vi "OFDM Symbol Type Mapper.vi"(9 "format":enum16{"NON_HT_OFDM", "VHT", "NON_HT_DUP_OFDM"}(ring), 10 "OFDM symbol index":u16) -> (2 "Cluster":T1)   [LabVIEW 2020]
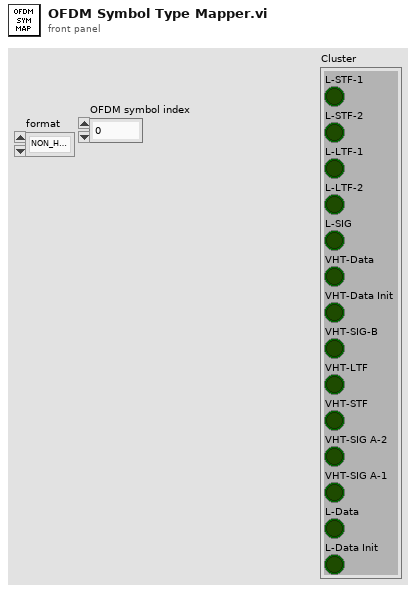
[diagram p1: front panel]
types:
  T1 = cluster{"L-STF-1":bool, "L-STF-2":bool, "L-LTF-1":bool, "L-LTF-2":bool, "L-SIG":bool, "VHT-Data":bool, "VHT-Data Init":bool, "VHT-SIG-B":bool, "VHT-LTF":bool, "VHT-STF":bool, "VHT-SIG A-2":bool, "VHT-SIG A-1":bool, "L-Data":bool, "L-Data Init":bool}
  T2 = enum16{"L-STF-1", "L-STF-2", "L-LTF-1", "L-LTF-2", "L-SIG", "L-Data-Init", "L-Data", "VHT-SIG A-1", "VHT-SIG A-2", "VHT-STF", "VHT-LTF", "VHT-SIG-B", "VHT-Data Init", "VHT-Data"}
  T3 = enum16{"L-STF-1", "L-STF-2", "L-LTF-1", "L-LTF-2", "L-SIG", "L-Data-Init", "L-Data", "VHT-SIG A-1", "VHT-SIG A-2", "VHT-STF", "VHT-LTF", "VHT-SIG-B", "VHT-Data Init", "VHT-Data"}[]
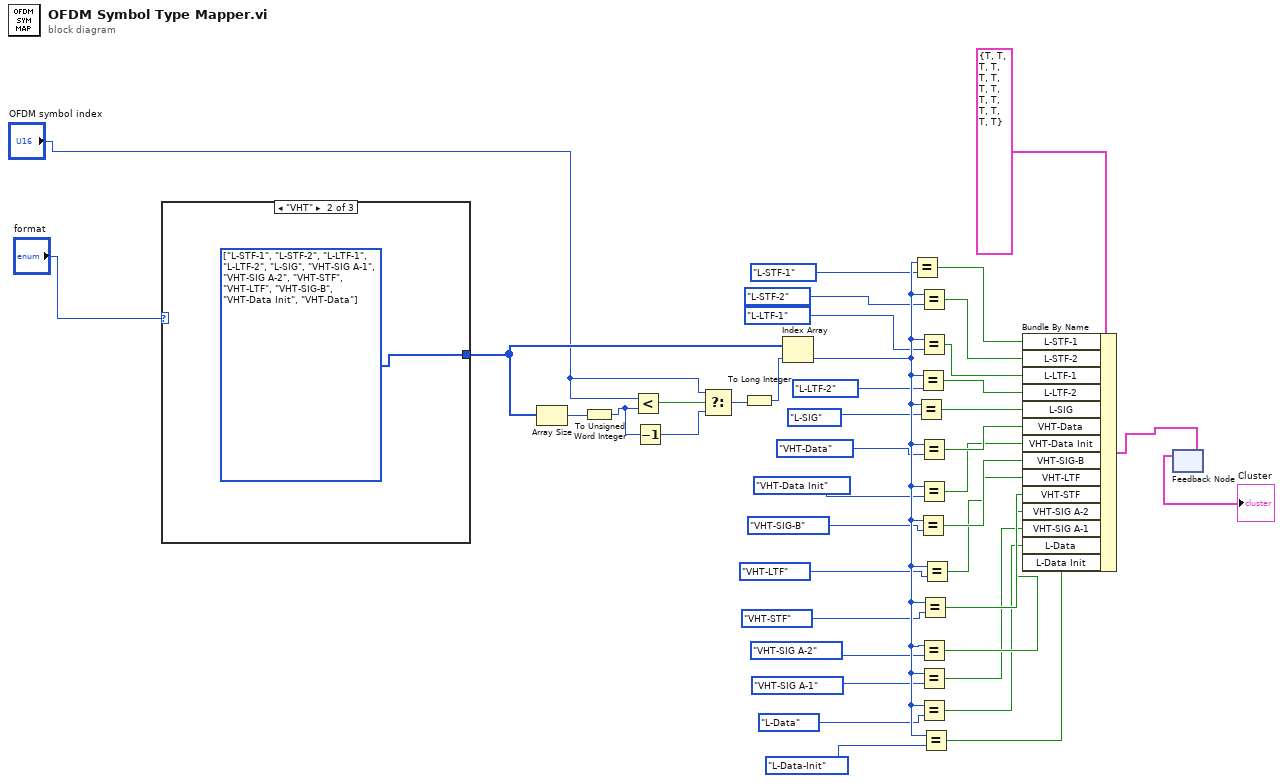
[diagram p0: block diagram]
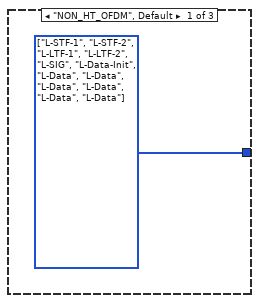
[diagram p2: hidden frame]
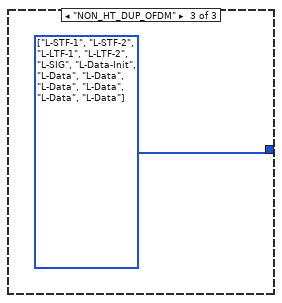
[diagram p3: hidden frame]
diagram:
  n1 = case shown="\"VHT\"" "format" {
    tunnel: [w42 w43 w44] -> w40
    frame "NON_HT_OFDM", Default {
      w42 = T3 [enum."L-STF-1", enum."L-STF-2", enum."L-LTF-1", enum."L-LTF-2", enum."L-SIG", enum."L-Data-Init", enum."L-Data", enum."L-Data", enum."L-Data", enum."L-Data", enum."L-Data", enum."L-Data"] items=["L-STF-1", "L-STF-2", "L-LTF-1", "L-LTF-2", "L-SIG", "L-Data-Init", "L-Data", "VHT-SIG A-1", "VHT-SIG A-2", "VHT-STF", "VHT-LTF", "VHT-SIG-B", "VHT-Data Init", "VHT-Data"]
    }
    frame "VHT" {
      w43 = T3 [enum."L-STF-1", enum."L-STF-2", enum."L-LTF-1", enum."L-LTF-2", enum."L-SIG", enum."VHT-SIG A-1", enum."VHT-SIG A-2", enum."VHT-STF", enum."VHT-LTF", enum."VHT-SIG-B", enum."VHT-Data Init", enum."VHT-Data"] items=["L-STF-1", "L-STF-2", "L-LTF-1", "L-LTF-2", "L-SIG", "L-Data-Init", "L-Data", "VHT-SIG A-1", "VHT-SIG A-2", "VHT-STF", "VHT-LTF", "VHT-SIG-B", "VHT-Data Init", "VHT-Data"]
    }
    frame "NON_HT_DUP_OFDM" {
      w44 = T3 [enum."L-STF-1", enum."L-STF-2", enum."L-LTF-1", enum."L-LTF-2", enum."L-SIG", enum."L-Data-Init", enum."L-Data", enum."L-Data", enum."L-Data", enum."L-Data", enum."L-Data", enum."L-Data"] items=["L-STF-1", "L-STF-2", "L-LTF-1", "L-LTF-2", "L-SIG", "L-Data-Init", "L-Data", "VHT-SIG A-1", "VHT-SIG A-2", "VHT-STF", "VHT-LTF", "VHT-SIG-B", "VHT-Data Init", "VHT-Data"]
    }
  }
  n2 = Array Size(array=w40) -> (size(s)=w39:i32)
  n3 = To Unsigned Word Integer(number=w39) -> (unsigned 16bit integer=w36:u16)
  n4 = Less?(x="OFDM symbol index", y=w36) -> (x < y?=w38:bool)
  n5 = Decrement(x=w36) -> (x-1=w35:u16)
  n6 = Select(t="OFDM symbol index", s=w38, f=w35) -> (s? t:f=w34:u16)
  n7 = To Long Integer(number=w34) -> (32bit integer=w33:i32)
  n8 = Index Array(array=w40, index=w33) -> (element=w32:T2)
  n9 = Equal?(x=w32, y=T2."L-STF-1") -> (x = y?=w16:bool)
  n10 = Equal?(x=w32, y=T2."L-SIG") -> (x = y?=w12:bool)
  n11 = Equal?(x=w32, y=T2."L-LTF-2") -> (x = y?=w13:bool)
  n12 = Equal?(x=w32, y=T2."VHT-SIG-B") -> (x = y?=w9:bool)
  n13 = Equal?(x=w32, y=T2."L-STF-2") -> (x = y?=w15:bool)
  n14 = Equal?(x=w32, y=T2."L-LTF-1") -> (x = y?=w14:bool)
  n15 = Equal?(x=w32, y=T2."VHT-Data") -> (x = y?=w11:bool)
  n16 = Equal?(x=w32, y=T2."VHT-Data Init") -> (x = y?=w10:bool)
  n17 = Equal?(x=w32, y=T2."VHT-SIG A-2") -> (x = y?=w6:bool)
  n18 = Equal?(x=w32, y=T2."VHT-SIG A-1") -> (x = y?=w5:bool)
  n19 = Equal?(x=w32, y=T2."L-Data") -> (x = y?=w4:bool)
  n20 = Equal?(x=w32, y=T2."VHT-STF") -> (x = y?=w7:bool)
  n21 = Equal?(x=w32, y=T2."L-Data-Init") -> (x = y?=w3:bool)
  n22 = Equal?(x=w32, y=T2."VHT-LTF") -> (x = y?=w8:bool)
  n23 = Bundle By Name(cluster=T1 {"L-STF-1"=TRUE, "L-STF-2"=TRUE, "L-LTF-1"=TRUE, "L-LTF-2"=TRUE, "L-SIG"=TRUE, "VHT-Data"=TRUE, "VHT-Data Init"=TRUE, "VHT-SIG-B"=TRUE, "VHT-LTF"=TRUE, "VHT-STF"=TRUE, "VHT-SIG A-2"=TRUE, "VHT-SIG A-1"=TRUE, "L-Data"=TRUE, "L-Data Init"=TRUE}, "L-STF-1"=w16, "L-STF-2"=w15, "L-LTF-1"=w14, "L-LTF-2"=w13, "L-SIG"=w12, "VHT-Data"=w11, "VHT-Data Init"=w10, "VHT-SIG-B"=w9, "VHT-LTF"=w8, "VHT-STF"=w7, "VHT-SIG A-2"=w6, "VHT-SIG A-1"=w5, "L-Data"=w4, "L-Data Init"=w3) -> (w2:T1)
  n24 = feedback-in #1(w2) -> ()
  n25 = feedback #1() -> (→"Cluster":T1)  [unwired: 1 in]
